vi "Biometry Average Keratometric Parameter2String.vi"(8 "error in (no error)":errorcluster caption="错误输入（无错误）", 9 "Biometry Average Standard Deviation":T1, 10 "Biometry Average State":T2, 11 "Biometry Average Parameter":T3) -> (0 "error out":errorcluster caption="错误输出", 2 "Data Output":string[][](array[string]))   [LabVIEW 2015, in "Utility VIs.lvlib"]
doc: "该模板用于创建子VI。"
uses:
  Utility VIs.lvlib
  Database Processing/Support/Table/Biometry Average Parameter.ctl
  Database Processing/Support/Table/Biometry Average State.ctl
  Database Processing/Support/Table/Biometry Average Standard Deviation.ctl
  Database Processing/Database Processing.lvlib
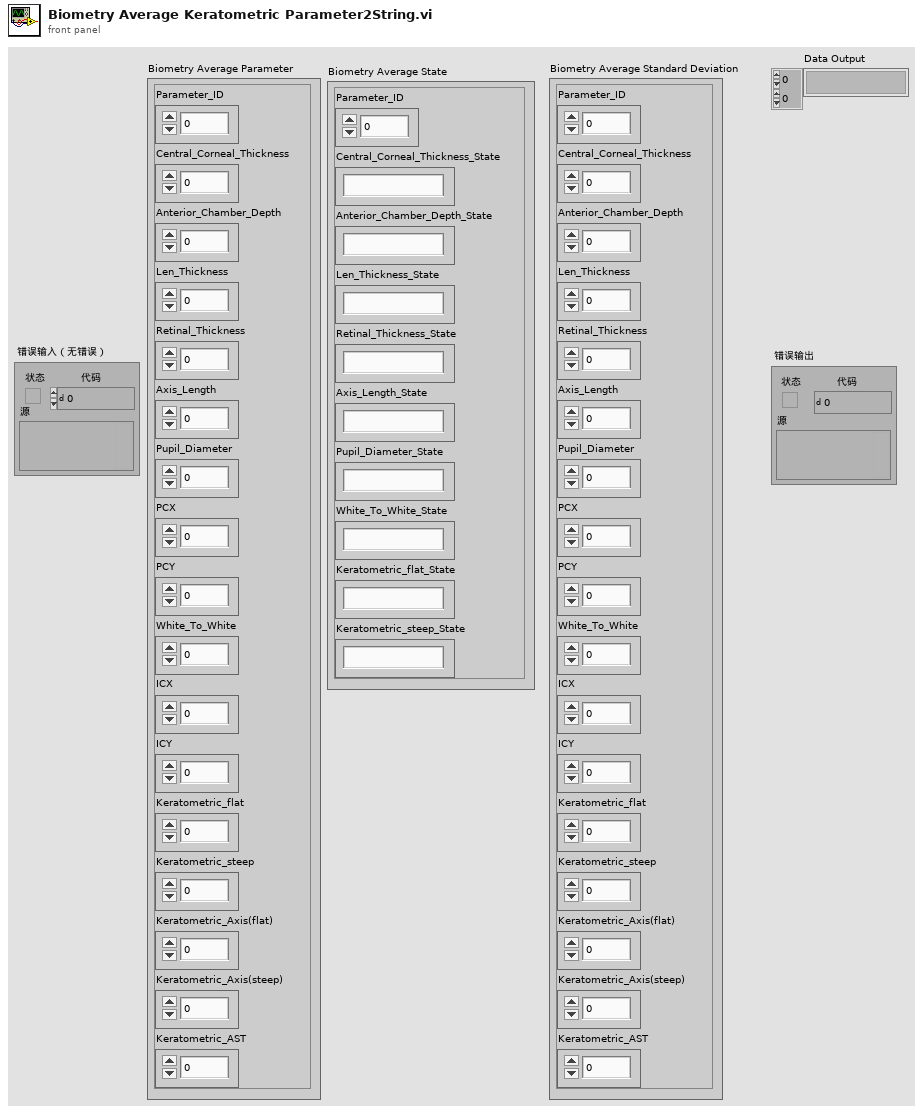
[diagram p1: front panel]
types:
  T1 = typedef "Database Processing.lvlib/Biometry Average Standard Deviation.ctl" = cluster{"Parameter_ID":i64, "Central_Corneal_Thickness":sgl, "Anterior_Chamber_Depth":sgl, "Len_Thickness":sgl, "Retinal_Thickness":sgl, "Axis_Length":sgl, "Pupil_Diameter":sgl, "PCX":sgl, "PCY":sgl, "White_To_White":sgl, "ICX":sgl, "ICY":sgl, "Keratometric_flat":sgl, "Keratometric_steep":sgl, "Keratometric_Axis(flat)":sgl, "Keratometric_Axis(steep)":sgl, "Keratometric_AST":sgl}
  T2 = typedef "Database Processing.lvlib/Biometry Average State.ctl" = cluster{"Parameter_ID":i64, "Central_Corneal_Thickness_State":string, "Anterior_Chamber_Depth_State":string, "Len_Thickness_State":string, "Retinal_Thickness_State":string, "Axis_Length_State":string, "Pupil_Diameter_State":string, "White_To_White_State":string, "Keratometric_flat_State":string, "Keratometric_steep_State":string}
  T3 = typedef "Database Processing.lvlib/Biometry Average Parameter.ctl" = cluster{"Parameter_ID":i64, "Central_Corneal_Thickness":sgl, "Anterior_Chamber_Depth":sgl, "Len_Thickness":sgl, "Retinal_Thickness":sgl, "Axis_Length":sgl, "Pupil_Diameter":sgl, "PCX":sgl, "PCY":sgl, "White_To_White":sgl, "ICX":sgl, "ICY":sgl, "Keratometric_flat":sgl, "Keratometric_steep":sgl, "Keratometric_Axis(flat)":sgl, "Keratometric_Axis(steep)":sgl, "Keratometric_AST":sgl}
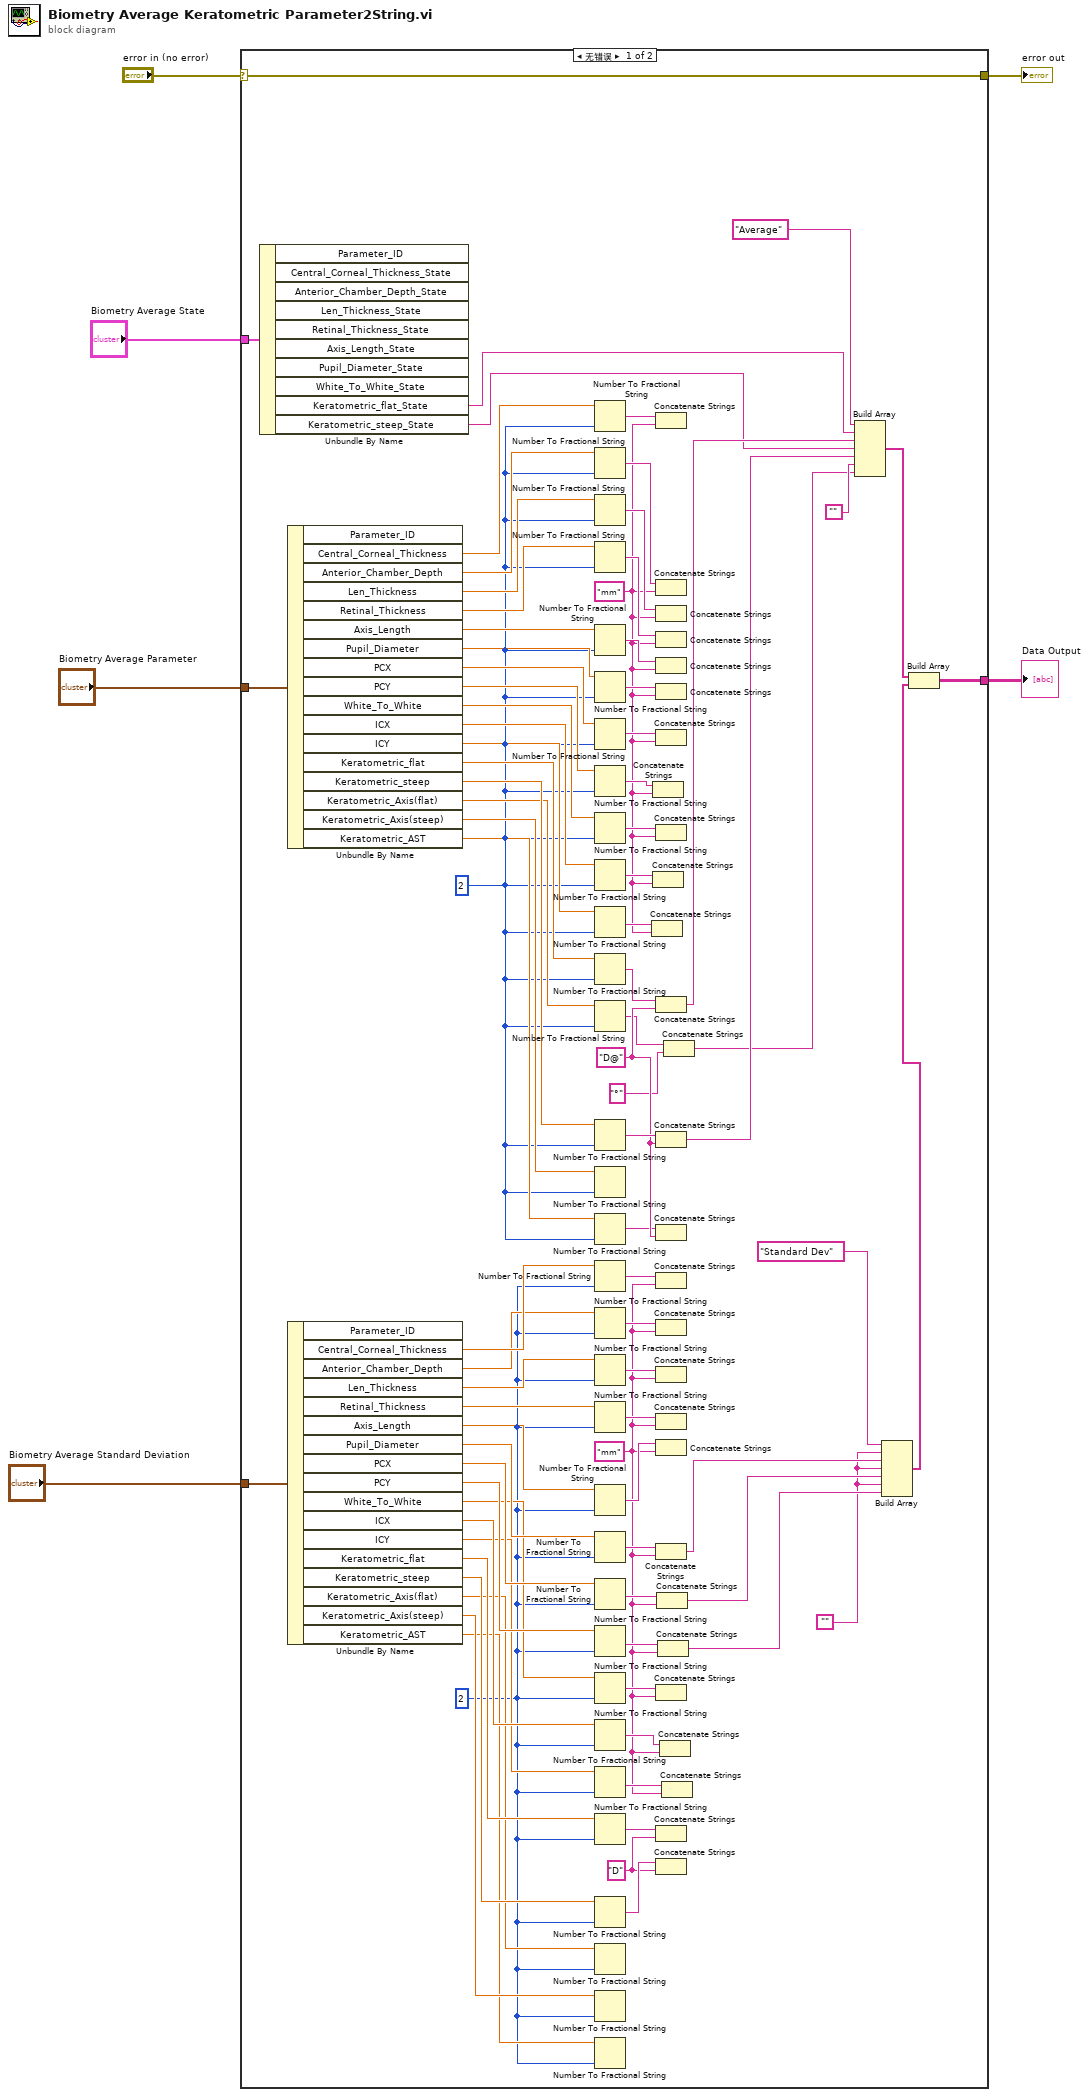
[diagram p0: block diagram]
diagram:
  n1 = case shown="无错误" "error in (no error)" {
    selector: "error in (no error)" -> [w36 w93]
    tunnel: [w36 w93] -> w5
    tunnel: "Biometry Average Parameter" -> [w92 _]
    tunnel: "Biometry Average Standard Deviation" -> [w91 _]
    tunnel: "Biometry Average State" -> [w90 _]
    tunnel: [w20 _] -> w1
    frame No Error {
      w14 = ""
      w37 = "D" ("字符串")
      w24 = "mm" ("字符串")
      w40 = i16 2 ("精度(6)")
      w30 = "D@" ("字符串")
      w31 = "mm" ("字符串")
      w50 = i16 2 ("精度(6)")
      n2 = Unbundle By Name(w90) -> ("Keratometric_flat_State"=w13:string, "Keratometric_steep_State"=w7:string)  [unwired: 8 out]
      n3 = Unbundle By Name(w92) -> ("Central_Corneal_Thickness"=w89:sgl, "Anterior_Chamber_Depth"=w88:sgl, "Len_Thickness"=w87:sgl, "Retinal_Thickness"=w86:sgl, "Axis_Length"=w85:sgl, "Pupil_Diameter"=w84:sgl, "PCX"=w83:sgl, "PCY"=w82:sgl, "White_To_White"=w81:sgl, "ICX"=w80:sgl, "ICY"=w79:sgl, "Keratometric_flat"=w78:sgl, "Keratometric_steep"=w77:sgl, "Keratometric_Axis(flat)"=w76:sgl, "Keratometric_Axis(steep)"=w52:sgl, "Keratometric_AST"=w51:sgl)  [unwired: 1 out]
      n4 = Unbundle By Name(w91) -> ("Central_Corneal_Thickness"=w75:sgl, "Anterior_Chamber_Depth"=w74:sgl, "Len_Thickness"=w73:sgl, "Retinal_Thickness"=w72:sgl, "Axis_Length"=w71:sgl, "Pupil_Diameter"=w70:sgl, "PCX"=w69:sgl, "PCY"=w68:sgl, "White_To_White"=w67:sgl, "ICX"=w66:sgl, "ICY"=w65:sgl, "Keratometric_flat"=w64:sgl, "Keratometric_steep"=w63:sgl, "Keratometric_Axis(flat)"=w62:sgl, "Keratometric_Axis(steep)"=w42:sgl, "Keratometric_AST"=w41:sgl)  [unwired: 1 out]
      n5 = Number To Fractional String(number=w89, precision (6)=w50) -> (F-format string=w61:string)  [unwired: 2 in]
      n6 = Number To Fractional String(number=w88, precision (6)=w50) -> (F-format string=w60:string)  [unwired: 2 in]
      n7 = Number To Fractional String(number=w87, precision (6)=w50) -> (F-format string=w59:string)  [unwired: 2 in]
      n8 = Number To Fractional String(number=w86, precision (6)=w50) -> (F-format string=w58:string)  [unwired: 2 in]
      n9 = Number To Fractional String(number=w85, precision (6)=w50) -> (F-format string=w57:string)  [unwired: 2 in]
      n10 = Number To Fractional String(number=w84, precision (6)=w50) -> (F-format string=w56:string)  [unwired: 2 in]
      n11 = Number To Fractional String(number=w83, precision (6)=w50) -> (F-format string=w35:string)  [unwired: 2 in]
      n12 = Number To Fractional String(number=w82, precision (6)=w50) -> (F-format string=w34:string)  [unwired: 2 in]
      n13 = Number To Fractional String(number=w81, precision (6)=w50) -> (F-format string=w55:string)  [unwired: 2 in]
      n14 = Number To Fractional String(number=w80, precision (6)=w50) -> (F-format string=w33:string)  [unwired: 2 in]
      n15 = Number To Fractional String(number=w79, precision (6)=w50) -> (F-format string=w32:string)  [unwired: 2 in]
      n16 = Number To Fractional String(number=w78, precision (6)=w50) -> (F-format string=w54:string)  [unwired: 2 in]
      n17 = Number To Fractional String(number=w76, precision (6)=w50) -> (F-format string=w10:string)  [unwired: 2 in]
      n18 = Number To Fractional String(number=w77, precision (6)=w50) -> (F-format string=w53:string)  [unwired: 2 in]
      n19 = Number To Fractional String(number=w52, precision (6)=w50) -> ()  [unwired: 2 in, 1 out]
      n20 = Number To Fractional String(number=w51, precision (6)=w50) -> (F-format string=w29:string)  [unwired: 2 in]
      n21 = Number To Fractional String(number=w75, precision (6)=w40) -> (F-format string=w49:string)  [unwired: 2 in]
      n22 = Number To Fractional String(number=w74, precision (6)=w40) -> (F-format string=w48:string)  [unwired: 2 in]
      n23 = Number To Fractional String(number=w73, precision (6)=w40) -> (F-format string=w47:string)  [unwired: 2 in]
      n24 = Number To Fractional String(number=w72, precision (6)=w40) -> (F-format string=w46:string)  [unwired: 2 in]
      n25 = Number To Fractional String(number=w71, precision (6)=w40) -> (F-format string=w45:string)  [unwired: 2 in]
      n26 = Number To Fractional String(number=w70, precision (6)=w40) -> (F-format string=w44:string)  [unwired: 2 in]
      n27 = Number To Fractional String(number=w69, precision (6)=w40) -> (F-format string=w28:string)  [unwired: 2 in]
      n28 = Number To Fractional String(number=w68, precision (6)=w40) -> (F-format string=w27:string)  [unwired: 2 in]
      n29 = Number To Fractional String(number=w67, precision (6)=w40) -> (F-format string=w43:string)  [unwired: 2 in]
      n30 = Number To Fractional String(number=w66, precision (6)=w40) -> (F-format string=w26:string)  [unwired: 2 in]
      n31 = Number To Fractional String(number=w65, precision (6)=w40) -> (F-format string=w25:string)  [unwired: 2 in]
      n32 = Number To Fractional String(number=w64, precision (6)=w40) -> (F-format string=w39:string)  [unwired: 2 in]
      n33 = Number To Fractional String(number=w63, precision (6)=w40) -> (F-format string=w38:string)  [unwired: 2 in]
      n34 = Number To Fractional String(number=w62, precision (6)=w40) -> ()  [unwired: 2 in, 1 out]
      n35 = Number To Fractional String(number=w42, precision (6)=w40) -> ()  [unwired: 2 in, 1 out]
      n36 = Number To Fractional String(number=w41, precision (6)=w40) -> ()  [unwired: 2 in, 1 out]
      n37 = Concatenate Strings(w32, w31) -> ()  [unwired: 1 out]
      n38 = Concatenate Strings(w34, w31) -> ()  [unwired: 1 out]
      n39 = Concatenate Strings(w33, w31) -> ()  [unwired: 1 out]
      n40 = Concatenate Strings(w61, w31) -> ()  [unwired: 1 out]
      n41 = Concatenate Strings(w60, w31) -> ()  [unwired: 1 out]
      n42 = Concatenate Strings(w59, w31) -> ()  [unwired: 1 out]
      n43 = Concatenate Strings(w58, w31) -> ()  [unwired: 1 out]
      n44 = Concatenate Strings(w57, w31) -> ()  [unwired: 1 out]
      n45 = Concatenate Strings(w56, w31) -> ()  [unwired: 1 out]
      n46 = Concatenate Strings(w35, w31) -> ()  [unwired: 1 out]
      n47 = Concatenate Strings(w55, w31) -> ()  [unwired: 1 out]
      n48 = Concatenate Strings(w54, w30) -> (w12:string)
      n49 = Concatenate Strings(w53, w30) -> (w11:string)
      n50 = Concatenate Strings(w29, w30) -> ()  [unwired: 1 out]
      n51 = Concatenate Strings(w49, w24) -> ()  [unwired: 1 out]
      n52 = Concatenate Strings(w48, w24) -> ()  [unwired: 1 out]
      n53 = Concatenate Strings(w47, w24) -> ()  [unwired: 1 out]
      n54 = Concatenate Strings(w46, w24) -> ()  [unwired: 1 out]
      n55 = Concatenate Strings(w45, w24) -> ()  [unwired: 1 out]
      n56 = Concatenate Strings(w44, w24) -> (w17:string)
      n57 = Concatenate Strings(w43, w24) -> ()  [unwired: 1 out]
      n58 = Concatenate Strings(w39, w37) -> ()  [unwired: 1 out]
      n59 = Concatenate Strings(w38, w37) -> ()  [unwired: 1 out]
      n60 = Concatenate Strings(w28, w24) -> (w16:string)
      n61 = Concatenate Strings(w27, w24) -> (w15:string)
      n62 = Concatenate Strings(w26, w24) -> ()  [unwired: 1 out]
      n63 = Concatenate Strings(w25, w24) -> ()  [unwired: 1 out]
      n64 = Concatenate Strings(w10, "°" ("字符串")) -> (w8:string)
      n65 = Build Array("Average" ("元素"), w13, w12, w7, w11, "", w8) -> (w22:string[])
      n66 = Build Array("Standard Dev" ("元素"), w14, w17, w14, w16, w14, w15) -> (w21:string[])
      n67 = Build Array(w22, w21) -> (w20:string[][])
    }
    frame Error {
    }
  }
  "error out" <- w5
  "Data Output" <- w1
